vi "GetDMMReference.vi"(4 "Session Name":string="SampleDMM") -> (0 "error out":errorcluster, 1 "Instrument Session":refnum<k7>)   [LabVIEW 2011]
doc: "This VI retrieves the session object that Session Name specifies and outputs the session object to TestStand. The session then exists for the \nlifetime of the execution."
uses:
  <vilib>/addons/TestStand/_SMUtility.llb/Session Manager - Get Instrument Session (32-bit).vi
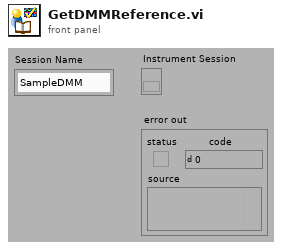
[diagram p1: front panel]
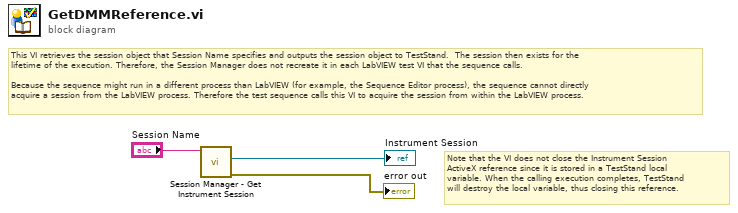
[diagram p0: block diagram]
diagram:
  # "Note that the VI does not close the Instrument Session\nActiveX reference since it is stored in a TestStand local\nvariable. When the calling execution completes, TestStand\nwill destroy the local variable, thus closing this reference."
  # "This VI retrieves the session object that Session Name specifies and outputs the session object to TestStand.  The session then exists for the \nlifetime of the execution. Therefore, the Session Manager does not recreate it in each LabVIEW test VI that the sequence calls.\n\nBecause the sequence might run in a different process than LabVIEW (for example, the Sequence Editor process), the sequence cannot directly\nacquire a session from the LabVIEW process. Therefore the test sequence calls this VI to acquire the session from within the LabVIEW process."
  n1 = call-poly <vilib>:"Session Manager - Get Instrument Session.vi"("Session Name"="Session Name") -> ("error out"=→"error out":errorcluster, "Instrument Session"=→"Instrument Session":refnum<k7>)  [unwired: 8 in, 1 out]
